vi "p72comprobacion.vi"() -> ()   [LabVIEW 2013]
panel:
  out "String":string="bulbasaur"
  out "Array":dbl[](array[numeric])
  in  "patrones":dbl[][](array[numeric])
  in  "path to BMP file":path
  in  "division":dbl[](array[numeric])=[0.1676082641555896, 0.0006470107597031312, 3.650732171329199e-05, 0.0005109250964092886, 9.1728578457172e-12, 3.832989546866887e-08, 2.1866027843027304e-11]
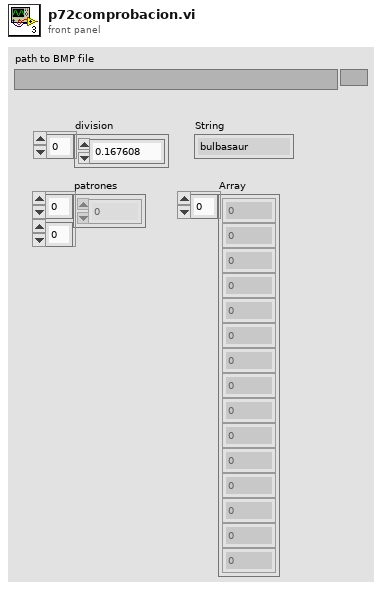
[diagram p1: front panel]
types:
  T1 = typedef "imagedata.ctl" = cluster{"image type":i32, "image depth":i32, "image":u8[], "mask":u8[], "colors":u32[], "Rectangle":cluster{"left":i16, "top":i16, "right":i16, "bottom":i16}}
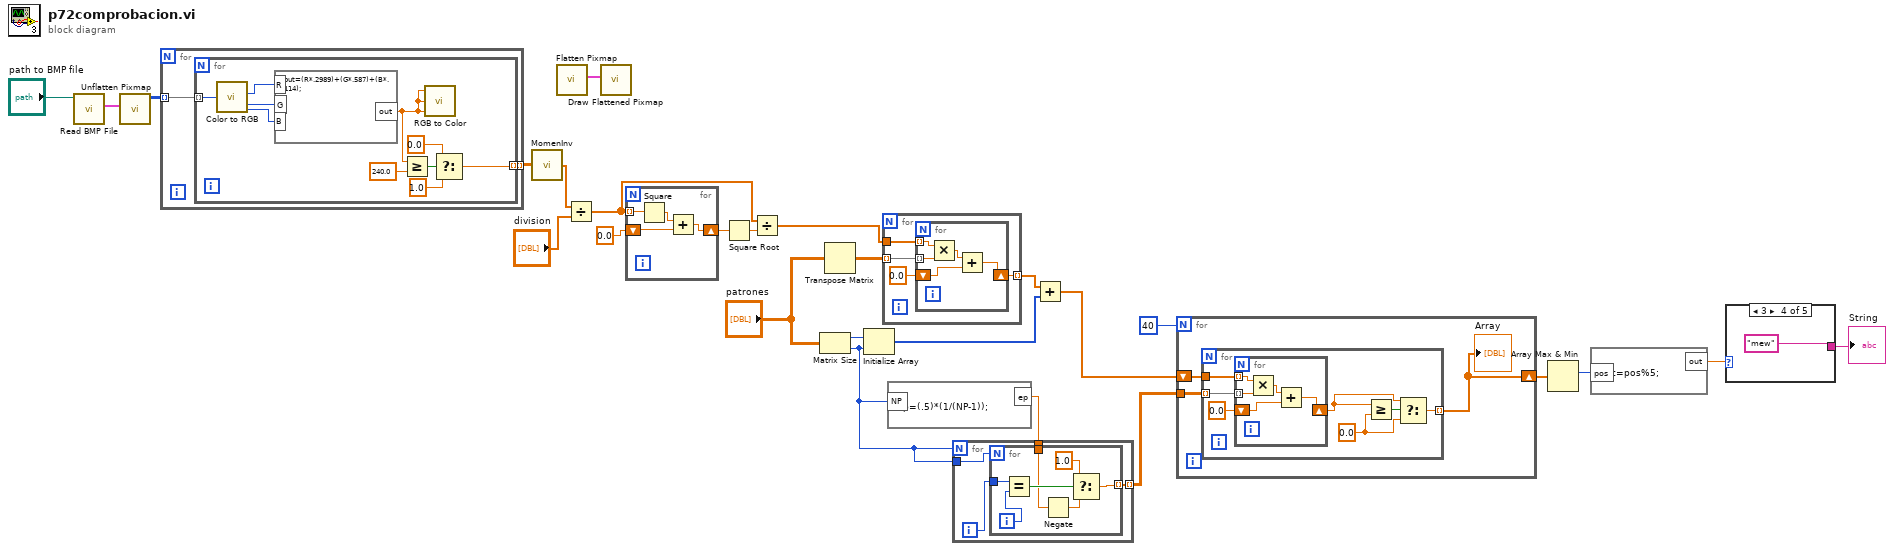
[diagram p0: block diagram]
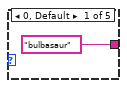
[diagram p2: hidden frame]
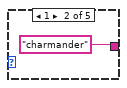
[diagram p3: hidden frame]
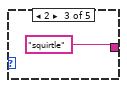
[diagram p4: hidden frame]
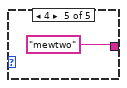
[diagram p5: hidden frame]
diagram:
  n1 = call <vilib>:"Read BMP File.vi"("path to BMP file"="path to BMP file") -> ("image data"=w25:T1)  [unwired: 8 in, 2 out]
  n2 = call <vilib>:"Unflatten Pixmap.vi"("image data"=w25) -> ("24-bit pixmap"=w24:u32[][])  [unwired: 4 in, 6 out]
  n3 = for {
    tunnel: w24 -> [w28] mode=indexing
    tunnel: [w27] -> w23 mode=indexing
    n4 = for {
      tunnel: w28 -> [w30] mode=indexing
      tunnel: [w29] -> w27 mode=indexing
      n5 = call <vilib>:"Color to RGB.vi"("Color"=w30) -> ("R"=w38:u8, "G"=w37:u8, "B"=w36:u8)  [unwired: 1 out]
      n6 = formula code="out=(R*.2989)+(G*.587)+(B*.114);"("R"=w38, "G"=w37, "B"=w36) -> ("out"=w31:dbl)
      n7 = Greater Or Equal?(x=w31, y=240.0) -> (x >= y?=w35:bool)
      n8 = call <vilib>:"RGB to Color.vi"("B"=w31, "G"=w31, "R"=w31) -> ()  [unwired: 1 out]
      n9 = Select(t=0.0, s=w35, f=1.0) -> (s? t:f=w29:dbl)
    }
  }
  n10 = call "MomenInv.vi"("Array 3"=w23) -> ("appended array"=w22:dbl[])
  n11 = call <vilib>:"Flatten Pixmap.vi"() -> ("image data"=w1:T1)  [unwired: 11 in]
  n12 = Divide(x=w22, y="division") -> (x/y=w17:dbl[])
  n13 = call <vilib>:"Draw Flattened Pixmap.vi"("image data"=w1) -> ()  [unwired: 8 in, 1 out]
  n14 = for {
    tunnel: w17 -> [w42] mode=indexing
    shift-right: [w39] -> w19
    shift-left: 0.0 -> [w40]
    n15 = Square(x=w42) -> (x^2=w41:dbl)
    n16 = Add(x=w41, y=w40) -> (x+y=w39:dbl)
  }
  n17 = Square Root(x=w19) -> (sqrt(x)=w18:dbl)
  n18 = Divide(x=w17, y=w18) -> (x/y=w13:dbl[])
  n19 = Matrix Size(0:"patrones") -> (1:w16:i32, 2:w10:i32)
  n20 = Transpose Matrix(1:"patrones") -> (0:w14:dbl[][])
  n21 = Initialize Array(w16, w10) -> (w11:i32[])
  n22 = for {
    tunnel: w14 -> [w46] mode=indexing
    tunnel: w13 -> [w45]
    tunnel: [w43] -> w12 mode=indexing
    n23 = for {
      tunnel: w46 -> [w51] mode=indexing
      tunnel: w45 -> [w50] mode=indexing
      shift-right: [w48] -> w43
      shift-left: 0.0 -> [w47]
      n24 = Multiply(x=w50, y=w51) -> (x*y=w49:dbl)
      n25 = Add(x=w49, y=w47) -> (x+y=w48:dbl)
    }
  }
  n26 = formula code="ep=(.5)*(1/(NP-1));"("NP"=w10) -> ("ep"=w9:dbl)
  n27 = for {
    N: w10 -> [_]
    tunnel: w10 -> [w54]
    tunnel: [w53] -> w7 mode=indexing
    tunnel: w9 -> [w52]
    i -> [w55]
    n28 = for {
      N: w54 -> [_]
      tunnel: w55 -> [w62]
      tunnel: [w58] -> w53 mode=indexing
      tunnel: w52 -> [w57]
      i -> [w61]
      n29 = Equal?(x=w62, y=w61) -> (x = y?=w60:bool)
      n30 = Negate(x=w57) -> (-x=w56:dbl)
      n31 = Select(t=1.0, s=w60, f=w56) -> (s? t:f=w58:dbl)
    }
  }
  n32 = Add(x=w12, y=w11) -> (x+y=w8:dbl[])
  n33 = for {
    N: 40 -> [_]
    tunnel: w7 -> [w64]
    shift-right: [w63] -> w6
    shift-left: w8 -> [w65]
    n34 = for {
      tunnel: w64 -> [w72] mode=indexing
      tunnel: w65 -> [w71]
      tunnel: [w69] -> w63 mode=indexing
      w66 = 0.0 ("y")
      n35 = for {
        tunnel: w72 -> [w77] mode=indexing
        tunnel: w71 -> [w76] mode=indexing
        shift-right: [w74] -> w67
        shift-left: 0.0 -> [w73]
        n36 = Multiply(x=w76, y=w77) -> (x*y=w75:dbl)
        n37 = Add(x=w75, y=w73) -> (x+y=w74:dbl)
      }
      n38 = Greater Or Equal?(x=w67, y=w66) -> (x >= y?=w68:bool)
      n39 = Select(t=w67, s=w68, f=w66) -> (s? t:f=w69:dbl)
    }
    "Array" <- w63
  }
  n40 = Array Max & Min(array=w6) -> (max index (indices)=w5:i32)  [unwired: 3 out]
  n41 = formula code="out=pos%5;"("pos"=w5) -> ("out"=w3:dbl)
  n42 = case shown="3" w3 {
    tunnel: ["bulbasaur" "charmander" "squirtle" "mew" "mewtwo"] -> w2
    frame 0, Default {
    }
    frame 1 {
    }
    frame 2 {
    }
    frame 3 {
    }
    frame 4 {
    }
  }
  "String" <- w2
